vi "Close Server.vi"(8 "error in (no error)":errorcluster, 11 "Server":refnum<class "Server.lvclass">) -> (0 "error out":errorcluster)   [LabVIEW 2020, in "Server.lvlib"]
doc: "Close the PVAccess server."
uses:
  Server.lvlib
  Server/Server.lvclass
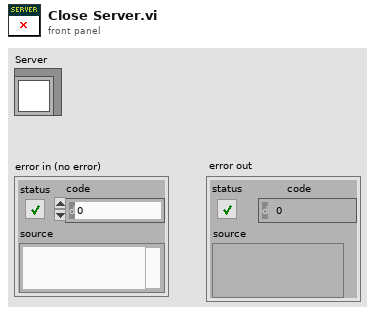
[diagram p1: front panel]
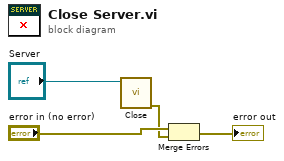
[diagram p0: block diagram]
diagram:
  n1 = call "Close.vi"("Server in"="Server") -> ("error out"=w2:errorcluster)  [unwired: 9 in, 1 out]
  n2 = Merge Errors("error in (no error)", w2) -> (→"error out":errorcluster)
